vi "启动.vi"() -> ()   [LabVIEW 2016]
uses:
  <vilib>/NI/Progress Bar/Controls/Update Bar Actions.ctl
  <vilib>/NI/Progress Bar/Controls/Progress Bar Properties.ctl
  <vilib>/NI/Progress Bar/Progress Bar.lvlib
  <vilib>/Utility/config.llb/NI_LVConfig.lvlib
panel:
  out "exists?":bool
  out "error out":errorcluster
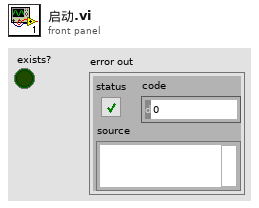
[diagram p1: front panel]
types:
  T1 = enum32{"Invalid", "Standard", "Closed", "Hidden", "Minimized", "Maximized"}
  T2 = typedef "Progress Bar.lvlib/Progress Bar Properties.ctl" = cluster{"Background Color":u32, "Installer Title":string, "Title Color":u32, "Action Text":string, "Text Color":u32, "Slider Value":u8, "Bar Color":u32, "Timeout":i32}
  T3 = typedef "Progress Bar.lvlib/Update Bar Actions.ctl" = enum16{"Add To Existing", "Set to Value"}
  T4 = typedef "NI_LVConfig.lvlib/Config Data RefNum.ctl" = refnum<k1>
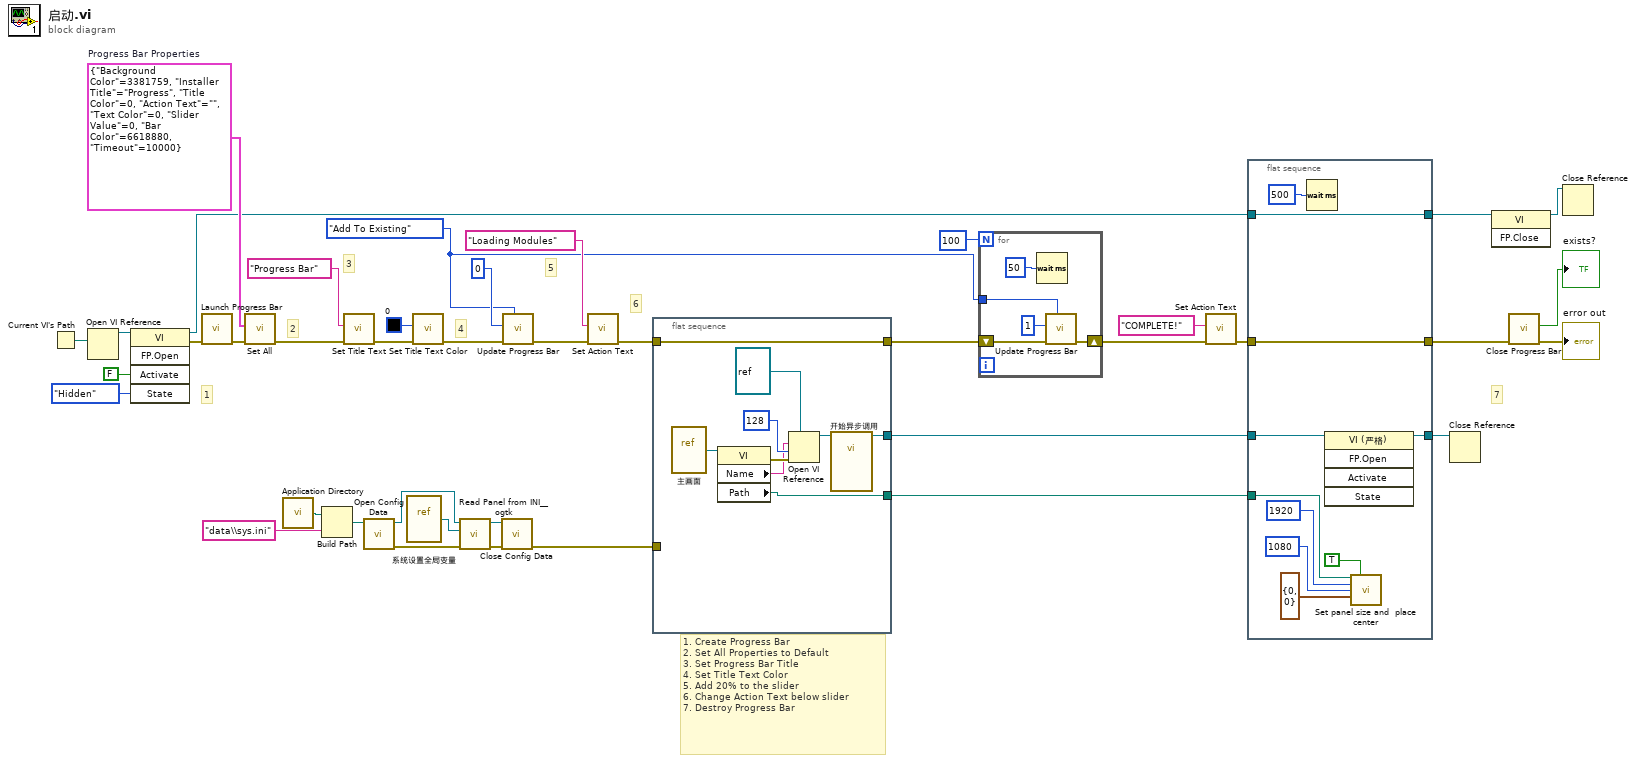
[diagram p0: block diagram]
diagram:
  w25 = T2 {"Background Color"=3381759, "Installer Title"="Progress", "Title Color"=0, "Action Text"="", "Text Color"=0, "Slider Value"=0, "Bar Color"=6618880, "Timeout"=10000}  # Progress Bar Properties
  w24 = Update_Bar_Actions."Add To Existing" ("Action")
  # "7"
  # "6"
  # "5"
  # "4"
  # "3"
  # "2"
  # "1"
  # "1. Create Progress Bar\n2. Set All Properties to Default\n3. Set Progress Bar Title\n4. Set Title Text Color\n5. Add 20% to the slider\n6. Change Action Text below slider\n7. Destroy Progress Bar"
  n1 = Current VI's Path() -> (path=w14:path)
  n2 = Open VI Reference(vi path=w14) -> (vi reference=w15:refnum<vi>)  [unwired: 5 in, 1 out]
  n3 = invoke class="VI" method="FP.Open"(reference=w15, "Activate"=FALSE ("激活？"), "State"=T1."Hidden" ("状态")) -> (reference out=w10:refnum<vi>, error out=w11:errorcluster)  [unwired: 2 in, 3 out]
  n4 = call <vilib>:"Launch Progress Bar.vi"("error in (no error)"=w11) -> ("error out"=w26:errorcluster)  [unwired: 9 in, 1 out]
  n5 = call <vilib>:"Set All.vi"("error in (no error)"=w26, "Progress Bar Properties (Default)"=w25) -> ("error out"=w36:errorcluster)  [unwired: 9 in]
  n6 = call <vilib>:"Application Directory.vi"() -> ("Application Directory"=w4:path)
  n7 = Build Path(base path=w4, name or relative path="data\\sys.ini" ("名称或相对路径")) -> (appended path=w2:path)
  n8 = call <vilib>:"Set Title Text.vi"("error in (no error)"=w36, "Installer Title"="Progress Bar") -> ("error out"=w39:errorcluster)  [unwired: 9 in]
  n9 = call <vilib>:"Open Config Data.vi"("configuration file path"=w2) -> ("error out"=w9:errorcluster, "refnum"=w8:T4)  [unwired: 8 in, 1 out]
  n10 = vi-ref "系统设置全局变量.vi"() -> (w7:refnum<vi>)
  n11 = call <vilib>:"Set Title Text Color.vi"("error in (no error)"=w39, "Color Box"=u32 0) -> ("error out"=w35:errorcluster)  [unwired: 9 in]
  n12 = call <userlib>:"Read Panel from INI__ogtk.vi"("error in (no error)"=w9, "VI ref"=w7, "refnum"=w8) -> ("error out"=w6:errorcluster, "refnum out"=w5:T4)  [unwired: 7 in]
  n13 = call <vilib>:"Close Config Data.vi"("error in (no error)"=w6, "refnum"=w5) -> ("error out"=w1:errorcluster)  [unwired: 8 in, 1 out]
  n14 = call <vilib>:"Update Progress Bar.vi"("Action"=w24, "error in (no error)"=w35, "Value"=u8 0) -> ("error out"=w34:errorcluster)  [unwired: 8 in]
  n15 = call <vilib>:"Set Action Text.vi"("error in (no error)"=w34, "Action Text"="Loading Modules") -> ("error out"=w33:errorcluster)  [unwired: 9 in]
  n16 = flat-sequence {
    tunnel: w33 -> [w49]
    tunnel: [w49] -> w31
    tunnel: [w48] -> w18
    tunnel: [w41] -> w16
    tunnel: w1 -> [_]
    frame #0 {
      n17 = vi-ref "主画面.vi"() -> (w43:refnum<vi>)
      n18 = property class="VI"(reference=w43) -> (error out=w47:errorcluster, "Name"=w44:string, "Path"=w41:path)  [unwired: 1 in, 1 out]
      n19 = Open VI Reference(type specifier VI Refnum (for type only)=refnum<vi> refnum ("类型说明符VI引用句柄（仅用于类型）"), vi path=w44, options=128 ("选项"), error in (no error)=w47) -> (vi reference=w42:refnum<vi>)  [unwired: 2 in, 1 out]
      n20 = call-by-ref "开始异步调用"(reference=w42) -> (reference out=w48:refnum<vi>)  [unwired: 13 in, 1 out]
    }
  }
  n21 = for {
    N: 100 ("Value") -> [_]
    tunnel: w24 -> [w51]
    shift-right: [w54] -> w30
    shift-left: w31 -> [w53]
    n22 = Wait (ms)(milliseconds to wait=u32 50) -> ()  [unwired: 1 out]
    n23 = call <vilib>:"Update Progress Bar.vi"("Action"=w51, "error in (no error)"=w53, "Value"=u8 1) -> ("error out"=w54:errorcluster)  [unwired: 8 in]
  }
  n24 = call <vilib>:"Set Action Text.vi"("error in (no error)"=w30, "Action Text"="COMPLETE!") -> ("error out"=w29:errorcluster)  [unwired: 9 in]
  n25 = flat-sequence {
    tunnel: w29 -> [w63]
    tunnel: [w63] -> w27
    tunnel: [w62] -> w19
    tunnel: w10 -> [w62]
    tunnel: w18 -> [w61]
    tunnel: [w60] -> w17
    tunnel: w16 -> [w55]
    frame #0 {
      n26 = Wait (ms)(milliseconds to wait=u32 500) -> ()  [unwired: 1 out]
      n27 = invoke class="VI (严格)" method="FP.Open"(reference=w61) -> (reference out=w60:refnum<vi>)  [unwired: 4 in, 4 out]
      n28 = call "Set panel size and  place center.vi"("Path"=w55, "Close Reference (false)"=TRUE, "Panel Width"=1920, "Panel Height"=1080, "FP.Origin in(H & V)"=cluster{"Horizontal":i16, "Vertical":i16} {"Horizontal"=0, "Vertical"=0}) -> ()  [unwired: 6 in, 5 out]
    }
  }
  n29 = Close Reference(reference=w17) -> ()  [unwired: 1 in, 1 out]
  n30 = invoke class="VI" method="FP.Close"(reference=w19) -> (reference out=w20:refnum<vi>)  [unwired: 2 in, 2 out]
  n31 = call <vilib>:"Close Progress Bar.vi"("error in (no error)"=w27) -> ("error out"=→"error out":errorcluster, "exists?"=→"exists?":bool)  [unwired: 9 in]
  n32 = Close Reference(reference=w20) -> ()  [unwired: 1 in, 1 out]
